vi "RemoveRefocus.vi"(7 "refocus_param":T1, 8 "triggers":u32[](array[numeric]), 11 "timetags":u32[](graph)) -> (0 "triggers":u32[](array[numeric]), 3 "timetags":u32[](graph))   [LabVIEW 2018]
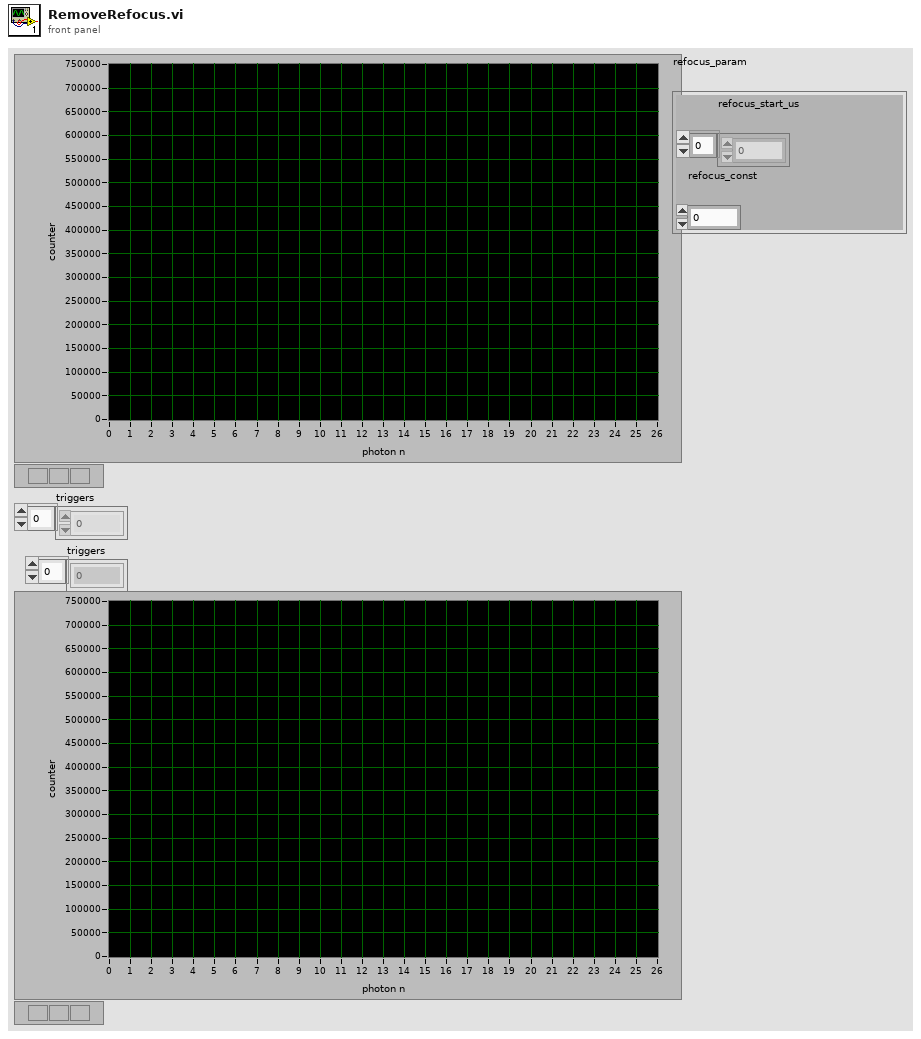
[diagram p1: front panel]
types:
  T1 = cluster{"refocus_start_us":u32[], "refocus_const":dbl}
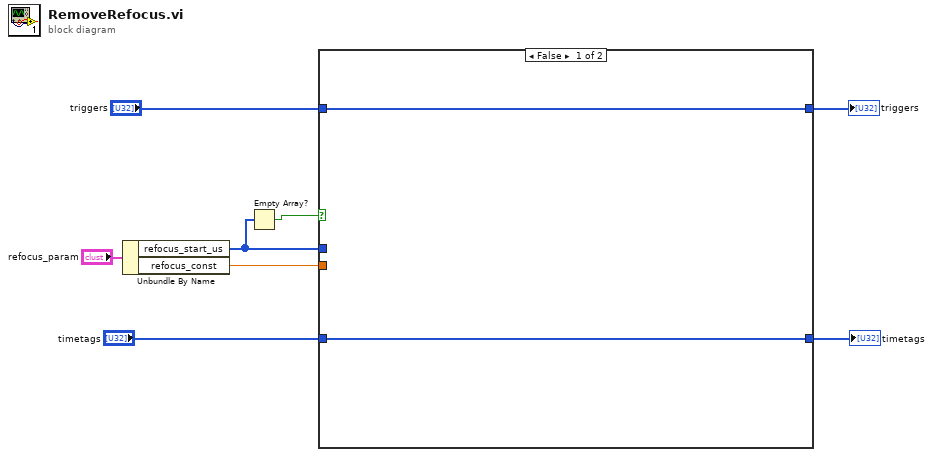
[diagram p0: block diagram]
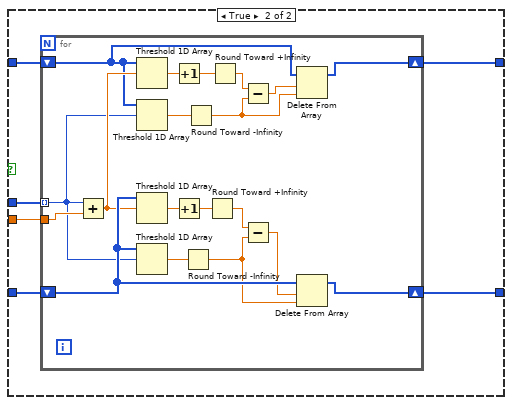
[diagram p2: hidden frame]
diagram:
  n1 = Unbundle By Name("refocus_param") -> ("refocus_start_us"=w4:u32[], "refocus_const"=w5:dbl)
  n2 = Empty Array?(array=w4) -> (empty?=w3:bool)
  n3 = case shown="False" w3 {
    tunnel: "timetags" -> [w10 w16]
    tunnel: "triggers" -> [w9 w15]
    tunnel: w4 -> [_ w14]
    tunnel: w5 -> [_ w13]
    tunnel: [w10 w12] -> w1
    tunnel: [w9 w11] -> w2
    frame False {
    }
    frame True {
      n4 = for {
        shift-right: [w27] -> w12
        shift-left: w16 -> [w30]
        shift-right: [w17] -> w11
        shift-left: w15 -> [w18]
        tunnel: w14 -> [w25] mode=indexing
        tunnel: w13 -> [w35]
        n5 = Add(x=w25, y=w35) -> (x+y=w26:dbl)
        n6 = Threshold 1D Array(2:w26, 3:w18) -> (0:w24:dbl)  [unwired: 1 in]
        n7 = Threshold 1D Array(2:w25, 3:w18) -> (0:w23:dbl)  [unwired: 1 in]
        n8 = Threshold 1D Array(2:w26, 3:w30) -> (0:w33:dbl)  [unwired: 1 in]
        n9 = Threshold 1D Array(2:w25, 3:w30) -> (0:w34:dbl)  [unwired: 1 in]
        n10 = Increment(x=w24) -> (x+1=w22:dbl)
        n11 = Increment(x=w33) -> (x+1=w32:dbl)
        n12 = Round Toward -Infinity(1:w34) -> (0:w29:dbl)
        n13 = Round Toward -Infinity(1:w23) -> (0:w19:dbl)
        n14 = Round Toward +Infinity(x=w32) -> (ceil(x): smallest int >= x=w31:dbl)
        n15 = Round Toward +Infinity(x=w22) -> (ceil(x): smallest int >= x=w21:dbl)
        n16 = Subtract(x=w21, y=w19) -> (x-y=w20:dbl)
        n17 = Subtract(x=w31, y=w29) -> (x-y=w28:dbl)
        n18 = Delete From Array(array=w18, length=w20, index=w19) -> (array with subset deleted=w17:u32[])  [unwired: 1 out]
        n19 = Delete From Array(array=w30, length=w28, index=w29) -> (array with subset deleted=w27:u32[])  [unwired: 1 out]
      }
    }
  }
  "triggers" <- w2
  "timetags" <- w1
